vi "_XNET Convert Time LV to U64 1ns.vi"(3 "Time LV":timestamp) -> (1 "Time U64 1ns":u64)   [LabVIEW 2018]
uses:
  nixlvapi.dll
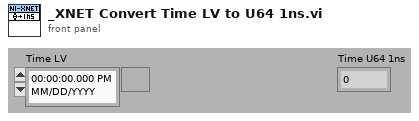
[diagram p1: front panel]
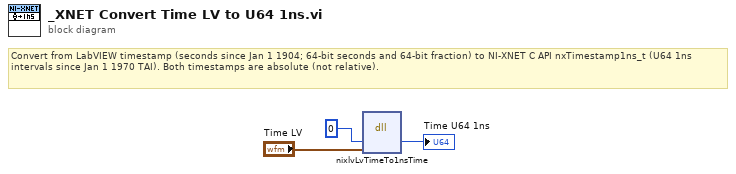
[diagram p0: block diagram]
diagram:
  # "Convert from LabVIEW timestamp (seconds since Jan 1 1904; 64-bit seconds and 64-bit fraction) to NI-XNET C API nxTimestamp1ns_t (U64 1ns intervals since Jan 1 1970 TAI). Both timestamps are absolute (not relative)."
  n1 = dll-call lib="nixlvapi.*" fn="nixlvLvTimeTo1nsTime" label="Call Library"("cTime"=u64 0 ("rawTime"), "lvTime"="Time LV") -> ("cTime"=→"Time U64 1ns":u64)  [unwired: 4 in, 3 out]
